vi "convert data type string to enum.vi"(8 "error in":errorcluster, 11 "Data Type String":string) -> (0 "error out":errorcluster, 3 "Data Type Enum":T1)   [LabVIEW 2013, in "fixed channel tag bus module configuration.lvclass"]
uses:
  fixed channel tag bus module configuration.lvclass
  <vilib>/NI/Tag Bus/tag/Data Type.ctl
  <vilib>/NI/Tag Bus/tag/tag descriptor.lvclass
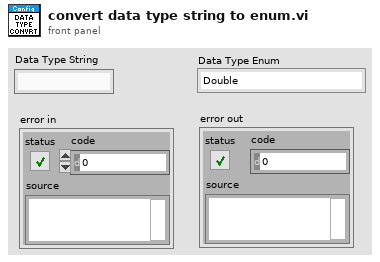
[diagram p1: front panel]
types:
  T1 = typedef "tag bus.lvlib/tag descriptor.lvclass/Data Type.ctl" = enum16{"Double", "Single", "I64", "I32", "I16", "I8", "U64", "U32", "U16", "U8", "Boolean", "String", "Array of Double", "Array of Single", "Array of I64", "Array of I32", "Array of I16", "Array of I8", "Array of U64", "Array of U32", "Array of U16", "Array of U8", "Array of Boolean", "Array of String"}
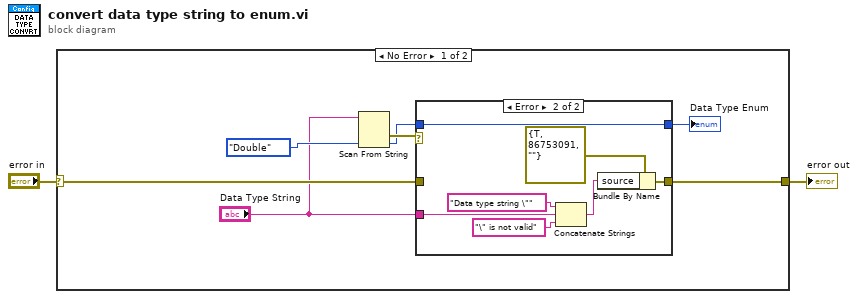
[diagram p0: block diagram]
diagram:
  n1 = case shown="No Error" "error in" {
    selector: "error in" -> [w8 w19]
    tunnel: [w7 w19] -> w1
    frame No Error {
      n2 = Scan From String(input string="Data Type String", default 1=Data_Type."Double" ("Data Type Enum 2")) -> (error out=w6:errorcluster, output 1=w3:T1)  [unwired: 3 in, 2 out]
      n3 = case shown="Error" w6 {
        tunnel: "Data Type String" -> [_ w16]
        tunnel: [w10 w13] -> w7
        tunnel: w3 -> [w11 w12]
        tunnel: [w11 w12] -> w9
        tunnel: w8 -> [w10 _]
        frame No Error {
        }
        frame Error {
          n4 = Concatenate Strings("Data type string \"" ("source"), w16, "\" is not valid" ("string")) -> (w14:string)
          n5 = Bundle By Name(cluster=errorcluster {"status"=TRUE, "code"=86753091, "source"=""} ("error constant"), "source"=w14) -> (w13:errorcluster)
        }
      }
      "Data Type Enum" <- w9
    }
    frame Error {
    }
  }
  "error out" <- w1
